vi "GetMeasureAt.vi"(10 "Sub Index":dbl[](array[numeric]), 11 "Measurement Data":i32[](array[numeric])) -> (2 "ir distances rf":dbl[][](array[numeric]), 3 "ir distances":dbl[](array[numeric]))   [LabVIEW 2016]
panel:
  out "XY Graph":cluster{dbl[], dbl[]}(graph)
  in  "Angel":dbl[](array[numeric])=[180.0, 135.0, 90.0]
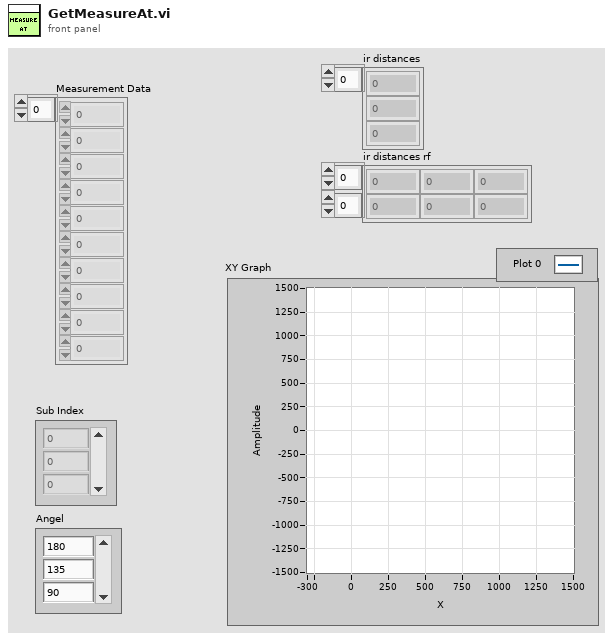
[diagram p1: front panel]
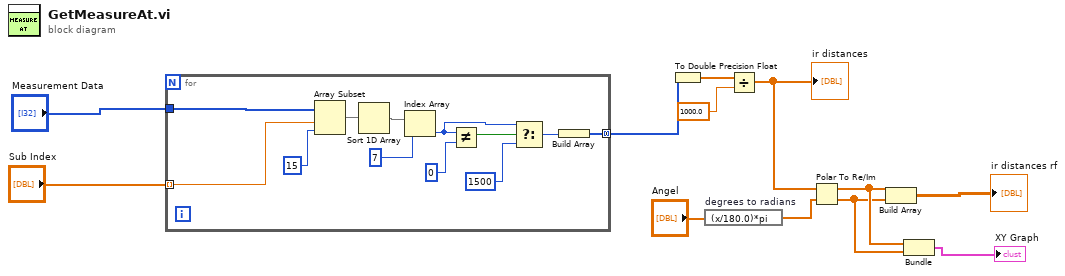
[diagram p0: block diagram]
diagram:
  n1 = for {
    tunnel: "Measurement Data" -> [w24]
    tunnel: "Sub Index" -> [w23] mode=indexing
    tunnel: [w18] -> w4 mode=concatenating
    n2 = Array Subset(array=w24, index=w23, length=15) -> (w21:i32[])
    n3 = Sort 1D Array(array=w21) -> (sorted array=w20:i32[])
    n4 = Index Array(array=w20, index=7) -> (element=w14:i32)
    n5 = Not Equal?(x=w14, y=0) -> (x != y?=w17:bool)
    n6 = Select(t=w14, s=w17, f=1500) -> (s? t:f=w15:i32)
    n7 = Build Array(w15) -> (w18:i32[])
  }
  n8 = To Double Precision Float(number=w4) -> (double precision float=w2:dbl[])
  n9 = expression code="(x/180.0)*pi" "degrees to radians"("Angel") -> (w9:dbl[])
  n10 = Divide(x=w2, y=1000.0) -> (x/y=w3:dbl[])
  "ir distances" <- w3
  n11 = Polar To Re/Im(2:w9, 3:w3) -> (0:w6:dbl[], 1:w7:dbl[])
  n12 = Build Array(w7, w6) -> (→"ir distances rf":dbl[][])
  n13 = Bundle(w7, w6) -> (→"XY Graph":cluster{dbl[], dbl[]})  [unwired: 1 in]
